vi "Beta 2.3.vi"() -> ()   [LabVIEW 2011]
uses:
  <vilib>/silver_ctls/ArrayMatrixCluster/Real Matrix NI_Silver.ctl
  <vilib>/vision/NI_Vision_Development_Module.lvlib
panel:
  in  "Real Matrix":T1
  in  "Morphology":u16(ring) items=["(none)", "AutoM", "Close", "Dilate", "Erode", "Gradient", "Open", "Thick", "Thin"]
  in  "Generate":bool
  in  "Look for":enum16{"Bright Objects", "Dark Objects"}(ring)
  in  "Method":T2(ring)=enum."Inter-class Variance"
  out "Binary":T3(plugin-control)
  out "Threshold Range":cluster{"Lower value":sgl, "Upper value":sgl}={"Lower value"=128.0, "Upper value"=255.0} {"Upper value" format="%.2f"; "Lower value" format="%.2f"}
  in  "Stop":bool
  in  "Browse":bool
  out "XY Graph":cluster{dbl[], dbl[]}(graph)
  out "Original Image":T3(plugin-control)
  out "Path to Image":path
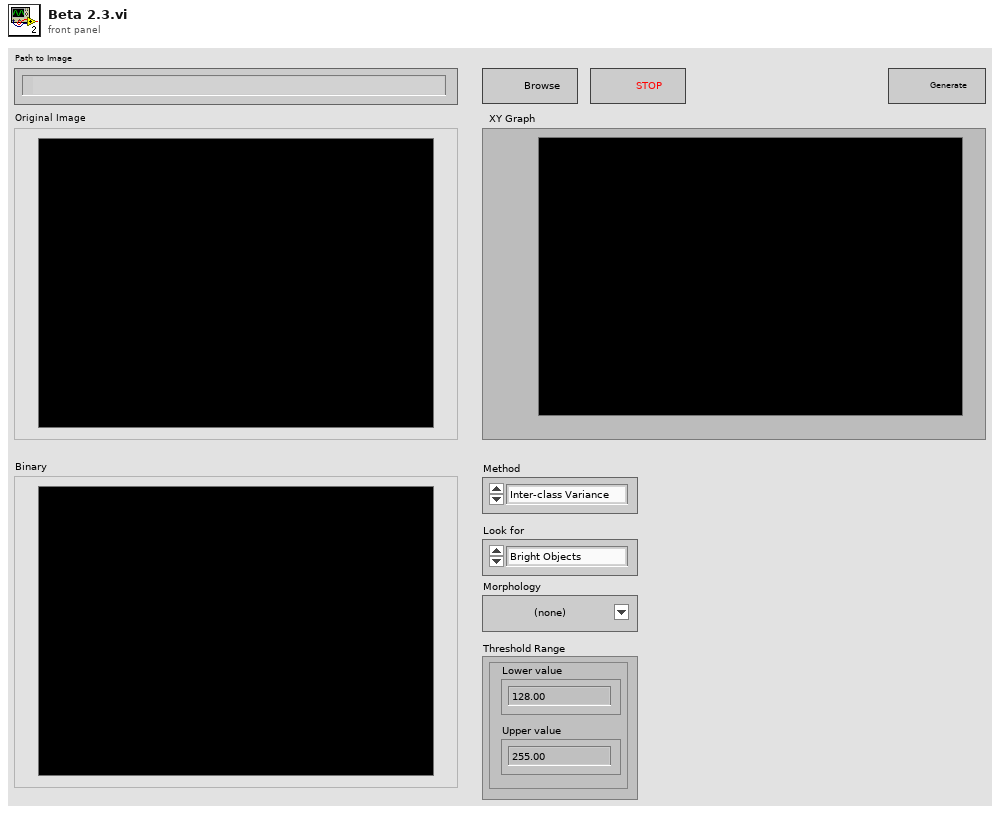
[diagram p1: front panel]
types:
  T1 = typedef "Real Matrix NI_Silver.ctl" = dbl[][]
  T2 = enum16{"Clustering", "Entropy", "Metric", "Moments", "Inter-class Variance"}
  T3 = typedef "IMAQ Image.ctl" = refnum<image>
  T4 = typedef "Image Type" = u32
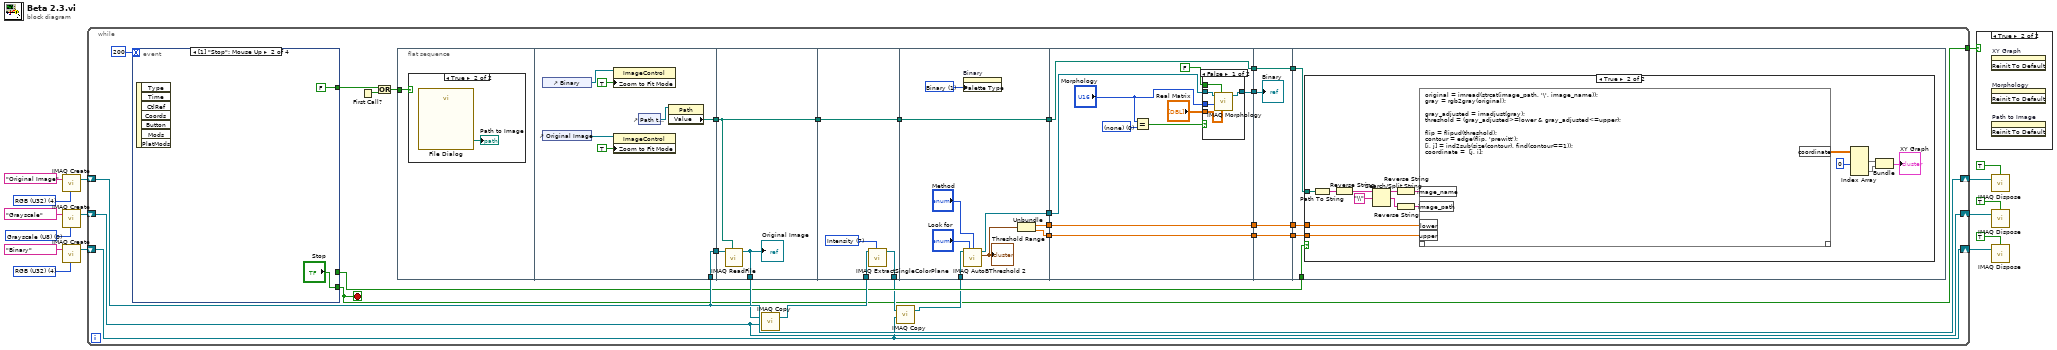
[diagram p0: block diagram]
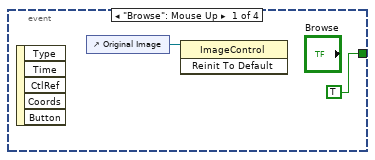
[diagram p3: hidden frame]
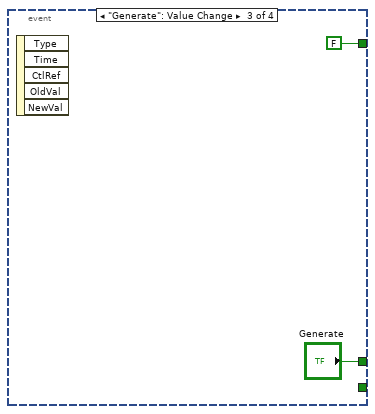
[diagram p4: hidden frame]
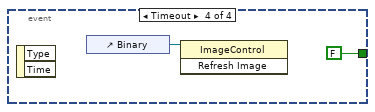
[diagram p5: hidden frame]
diagram:
  w4 = T4 4 items=["Grayscale (U8)", "Grayscale (I16)", "Grayscale (SGL)", "Complex (CSG)", "RGB (U32)", "HSL (U32)", "RGB (U64)", "Grayscale (U16)"] ("Image Type")
  w10 = T4 0 items=["Grayscale (U8)", "Grayscale (I16)", "Grayscale (SGL)", "Complex (CSG)", "RGB (U32)", "HSL (U32)", "RGB (U64)", "Grayscale (U16)"] ("Image Type")
  w15 = T4 4 items=["Grayscale (U8)", "Grayscale (I16)", "Grayscale (SGL)", "Complex (CSG)", "RGB (U32)", "HSL (U32)", "RGB (U64)", "Grayscale (U16)"] ("Image Type")
  n1 = call "IMAQ Create"("Image Name"="Original Image", "Image Type"=w15) -> ("New Image"=w14:T3)  [unwired: 3 in, 1 out]
  n2 = call "IMAQ Create"("Image Name"="Grayscale", "Image Type"=w10) -> ("New Image"=w9:T3)  [unwired: 3 in, 1 out]
  n3 = call "IMAQ Create"("Image Name"="Binary", "Image Type"=w4) -> ("New Image"=w1:T3)  [unwired: 3 in, 1 out]
  n4 = while {
    shift-right: [w39] -> w13
    shift-left: w14 -> [w39]
    tunnel: [w17] -> w12
    shift-right: [w33] -> w7
    shift-left: w9 -> [w33]
    shift-right: [w27] -> w2
    shift-left: w1 -> [w27]
    stop <- w17 stop-if-true
    n5 = event shown="[1] \"Stop\": Mouse Up" {
      selector: _ -> [_ _ _ _]
      dyn-events: _ -> [_ _ _ _]
      timeout: 200 -> [_ _ _ _]
      tunnel: [TRUE FALSE FALSE FALSE] -> w43
      tunnel: [_ "Stop" _ _] -> w17
      tunnel: [_ _ "Generate" _] -> w32
      event "Browse": Mouse Up {
        n6 = event-data() -> ()  [unwired: 1 in, 5 out]
        n7 = control-ref of="Original Image"() -> (w46:refnum<vi>)
        n8 = invoke class="ImageControl" method="Reinit To Default"(reference=w46) -> ()  [unwired: 2 in, 3 out]
      }
      event "Stop": Mouse Up {
        n9 = event-data() -> ()  [unwired: 1 in, 7 out]
      }
      event "Generate": Value Change {
        n10 = event-data() -> ()  [unwired: 1 in, 5 out]
      }
      event Timeout {
        n11 = event-data() -> ()  [unwired: 1 in, 2 out]
        n12 = control-ref of="Binary"() -> (w52:refnum<vi>)
        n13 = invoke class="ImageControl" method="Refresh Image"(reference=w52) -> ()  [unwired: 2 in, 3 out]
      }
    }
    n14 = First Call?() -> (First Call?: T/F=w42:bool)
    n15 = Or(x=w43, y=w42) -> (x .or. y?=w41:bool)
    n16 = flat-sequence {
      tunnel: w41 -> [w53]
      tunnel: [w57] -> w44
      tunnel: [w58] -> w40
      tunnel: w39 -> [w57]
      tunnel: w44 -> [w63]
      tunnel: w40 -> [w64]
      tunnel: [w64] -> w38
      tunnel: [w62] -> w35
      tunnel: w38 -> [w68]
      tunnel: [w68] -> w37
      tunnel: w34 -> [w66]
      tunnel: [w65] -> w28
      tunnel: w37 -> [w77]
      tunnel: [w77] -> w25
      tunnel: [w76] -> w23
      tunnel: [w71] -> w22
      tunnel: [w70] -> w20
      tunnel: w29 -> [w69]
      tunnel: w25 -> [w87]
      tunnel: [w87] -> w24
      tunnel: w23 -> [w84]
      tunnel: w22 -> [w86]
      tunnel: [w86] -> w21
      tunnel: w20 -> [w85]
      tunnel: [w85] -> w19
      tunnel: [w83] -> w18
      tunnel: w24 -> [w97]
      tunnel: [w97] -> w36
      tunnel: [w96] -> w31
      tunnel: w21 -> [w96]
      tunnel: [w95] -> w30
      tunnel: w19 -> [w95]
      tunnel: w18 -> [w94]
      tunnel: w36 -> [w101]
      tunnel: w32 -> [w100]
      tunnel: w31 -> [w99]
      tunnel: w30 -> [w98]
      frame #0 {
        n17 = case shown="True" w53 {
          frame False {
          }
          frame True {
            n18 = call "File Dialog"() -> ("selected path"=→"Path to Image":path)  [unwired: 12 in, 3 out]
          }
        }
      }
      frame #1 {
        n19 = control-ref of="Binary"() -> (w56:refnum<vi>)
        n20 = control-ref of="Original Image"() -> (w61:refnum<vi>)
        n21 = property class="ImageControl"(reference=w56, "Zoom to Fit Mode"=TRUE) -> ()  [unwired: 1 in, 2 out]
        n22 = property class="ImageControl"(reference=w61, "Zoom to Fit Mode"=TRUE) -> ()  [unwired: 1 in, 2 out]
        n23 = control-ref of="Path to Image"() -> (w59:refnum<vi>)
        n24 = property class="Path"(reference=w59) -> ("Value"=w58:path)  [unwired: 1 in, 2 out]
      }
      frame #2 {
        n25 = call "IMAQ ReadFile"("File Path"=w64, "Image"=w63) -> ("Image Out"=w62:T3)  [unwired: 5 in, 4 out]
        "Original Image" <- w62
      }
      frame #3 {
        w67 = 7 items=["Red", "Green", "Blue", "Hue", "Saturation", "Luminance", "Value", "Intensity"] ("Color Plane")
        n26 = call "IMAQ ExtractSingleColorPlane"("Color Plane"=w67, "Image Src"=w66) -> ("Image Dst Out"=w65:T3)  [unwired: 8 in, 1 out]
      }
      frame #4 {
        w75 = u32 1 items=["Grayscale", "Binary", "Gradient", "Rainbow", "Temperature", "User Defined"] ("Palette")
        n27 = property on="Binary" class="ImageControl"("Palette Type"=w75) -> ()  [unwired: 2 in, 2 out]
        n28 = call "IMAQ AutoBThreshold 2"("Image Src"=w69, "Look For (Bright Objects)"="Look for", "Method (clustering)"="Method") -> ("Image Dst Out"=w76:T3, "Threshold Range Out"=w72:cluster{"Lower value":sgl, "Upper value":sgl})  [unwired: 10 in, 1 out]
        "Threshold Range" <- w72
        n29 = Unbundle(w72) -> ("Lower value"=w71:sgl, "Upper value"=w70:sgl)
      }
      frame #5 {
        w80 = u16 0 items=["(none)"]
        n30 = Equal?(x="Morphology", y=w80) -> (x = y?=w79:bool)
        n31 = case shown="False" w79 {
          tunnel: w84 -> [w88 w93]
          tunnel: [w89 w93] -> w83
          tunnel: FALSE -> [w91 _]
          tunnel: "Real Matrix" -> [w90 _]
          tunnel: "Morphology" -> [w92 _]
          frame False {
            n32 = call "IMAQ Morphology"("Structuring Element"=w90, "Square/Hexa (Square)"=w91, "Operation"=w92, "Image Src"=w88) -> ("Image Dst Out"=w89:T3)  [unwired: 6 in, 1 out]
          }
          frame True {
          }
        }
      }
      frame #6 {
        "Binary" <- w94
      }
      frame #7 {
        n33 = case shown="True" w100 {
          tunnel: w101 -> [_ w116]
          tunnel: w99 -> [_ w103]
          tunnel: w98 -> [_ w102]
          frame False {
          }
          frame True {
            n34 = Path To String(path=w116) -> (string=w115:string)
            n35 = Reverse String(1:w115) -> (0:w114:string)
            n36 = Search/Split String(string=w114, search string/char (-)="\\") -> (substring before match=w112:string, match + rest of string=w111:string)  [unwired: 1 in, 1 out]
            n37 = Reverse String(1:w112) -> (0:w110:string)
            n38 = Reverse String(1:w111) -> (0:w109:string)
            n39 = script code="original = imread(strcat(image_path, '\\', image_name));\ngray = rgb2gray(original);\n\ngray_adjusted = imadjust(gray);\nthreshold = (gray_adjusted>=lower & gray_adjusted<=upper);\n\nflip = flipud(threshold);\ncontour = edge(flip, 'prewitt');\n[i, j] = ind2sub(size(contour), find(contour==1));\ncoordinate =  [j, i];"("image_name"=w110, "image_path"=w109, "lower"=w103, "upper"=w102) -> ("coordinate"=w108:dbl[][])  [unwired: 1 in, 1 out]
            n40 = Index Array(array=w108, index (col) #1=0 ("disabled index (col)")) -> (element #1=w107:dbl[], element #2=w106:dbl[])  [unwired: 3 in]
            n41 = Bundle(w107, w106) -> (→"XY Graph":cluster{dbl[], dbl[]})  [unwired: 1 in]
          }
        }
      }
    }
    n42 = call "IMAQ Copy"("Image Dst"=w33, "Image Src"=w35) -> ("Image Dst Out"=w34:T3)  [unwired: 4 in, 1 out]
    n43 = call "IMAQ Copy"("Image Dst"=w27, "Image Src"=w28) -> ("Image Dst Out"=w29:T3)  [unwired: 4 in, 1 out]
  }
  n44 = case shown="True" w12 {
    frame False {
    }
    frame True {
      n45 = invoke on="XY Graph" class="XYGraph (strict)" method="Reinit To Default"() -> ()  [unwired: 3 in, 3 out]
      n46 = invoke on="Morphology" class="Ring (strict)" method="Reinit To Default"() -> ()  [unwired: 3 in, 3 out]
      n47 = invoke on="Path to Image" class="Path" method="Reinit To Default"() -> ()  [unwired: 3 in, 3 out]
    }
  }
  n48 = call "IMAQ Dispose"("All Images? (No)"=TRUE, "Image"=w13) -> ()  [unwired: 4 in, 1 out]
  n49 = call "IMAQ Dispose"("All Images? (No)"=TRUE, "Image"=w7) -> ()  [unwired: 4 in, 1 out]
  n50 = call "IMAQ Dispose"("All Images? (No)"=TRUE, "Image"=w2) -> ()  [unwired: 4 in, 1 out]
